vi "_Main.vi"   [LabVIEW 2017, in "Drive.lvlib"]
uses:
  Drive.lvlib
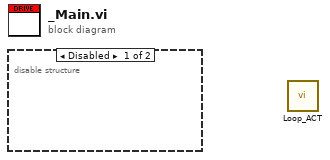
[diagram p0: block diagram]
diagram:
  n1 = disable-structure shown="Disabled" {
    frame Disabled {
    }
    frame Enabled {
    }
  }
  n2 = call "Loop_ACT.vi"() -> ()  [unwired: 12 in]
